vi "subviM_P.vi"(1 "PARO in":bool, 2 "MARCHA in":bool) -> (0 "Boolean":bool)   [LabVIEW 2020]
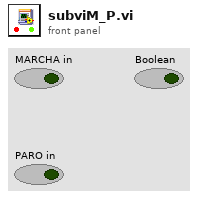
[diagram p1: front panel]
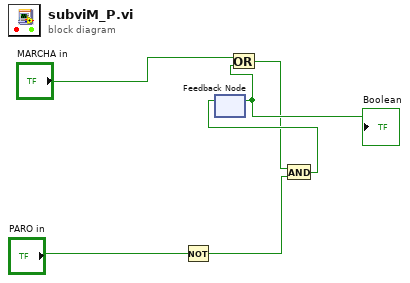
[diagram p0: block diagram]
diagram:
  n1 = Not(x="PARO in") -> (.not. x?=w4:bool)
  n2 = feedback #1() -> (w6:bool)  [unwired: 1 in]
  "Boolean" <- w6
  n3 = Or(x="MARCHA in", y=w6) -> (x .or. y?=w2:bool)
  n4 = And(x=w2, y=w4) -> (x .and. y?=w5:bool)
  n5 = feedback-in #1(w5) -> ()
